vi "angleToDist.vi"(8 "y":dbl=1.0 format="%#_13g", 9 "angle":dbl=60.0 format="%#_13g", 10 "y":dbl=1.0 format="%#_13g", 11 "x":dbl=1.732 format="%#_13g") -> (0 "tan(x)":dbl, 3 "angle":dbl)   [LabVIEW 2015]
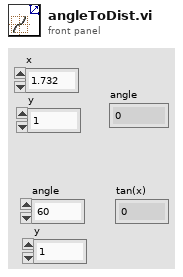
[diagram p1: front panel]
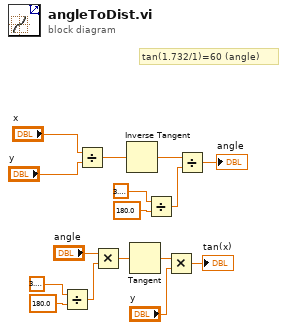
[diagram p0: block diagram]
diagram:
  # "tan(1.732/1)=60 (angle)"
  n1 = Divide(x=3.141592653589793, y=180.0) -> (x/y=w5:dbl)
  n2 = Divide(x="x", y="y") -> (x/y=w14:dbl)
  n3 = Multiply(x="angle", y=w5) -> (x*y=w4:dbl)
  n4 = Inverse Tangent(1:w14) -> (0:w13:dbl)
  n5 = Tangent(1:w4) -> (0:w3:dbl)
  n6 = Divide(x=3.141592653589793, y=180.0) -> (x/y=w9:dbl)
  n7 = Multiply(x=w3, y="y") -> (x*y=→"tan(x)":dbl)
  n8 = Divide(x=w13, y=w9) -> (x/y=→"angle":dbl)
